vi "Create Arbitrary Waveform.vi"(6 "Arbitrary Numeric Waveform Data":dbl[](array[numeric])=[1000.0, 2000.0, 3000.0, 4000.0, 5000.0, 6000.0, 7000.0, 8000.0], 7 "Waveform Parameters":T1={"Frequency (1000 Hz)"=1000.0, "Amplitude (2.0 Vpp)"=2.0, "DC Offset (0.00 V)"=0.0, "Phase (0.0 degrees)"=0.002} {"Phase (0.0 degrees)" min=-360.0 max=360.0 format="%#.1g"; "DC Offset (0.00 V)" min=-10.0 max=10.0; "Amplitude (2.0 Vpp)" min=0.001 max=20.0 step=1.0 format="%#.3f"; "Frequency (1000 Hz)" min=1e-06 max=160000000.0 step=1.0 format="%#.6g"}, 8 "error in (no error)":errorcluster, 9 "Select Channel (1:Channel 1)":i32(ring)=1 items=["Channel 1"=1, "Channel 2"=2], 10 "Waveform Name (\"wave1\")":string="wave1", 11 "VISA resource name":refnum<visa-resource-name>) -> (0 "error out":errorcluster, 3 "VISA resource name out":refnum<visa-resource-name>)   [LabVIEW 2023, in "Siglent SDG X Series.lvlib"]
doc: "Creates and saves an arbitrary (user-defined) waveform in non-volatile memory, then selects it for output."
uses:
  Siglent SDG X Series.lvlib
  <vilib>/Utility/error.llb/Trim Whitespace One-Sided.vi
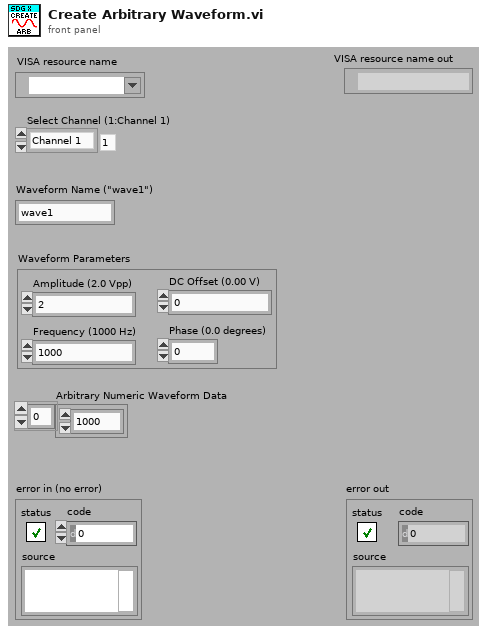
[diagram p1: front panel]
types:
  T1 = cluster{"Frequency (1000 Hz)":dbl, "Amplitude (2.0 Vpp)":dbl, "DC Offset (0.00 V)":dbl, "Phase (0.0 degrees)":dbl}
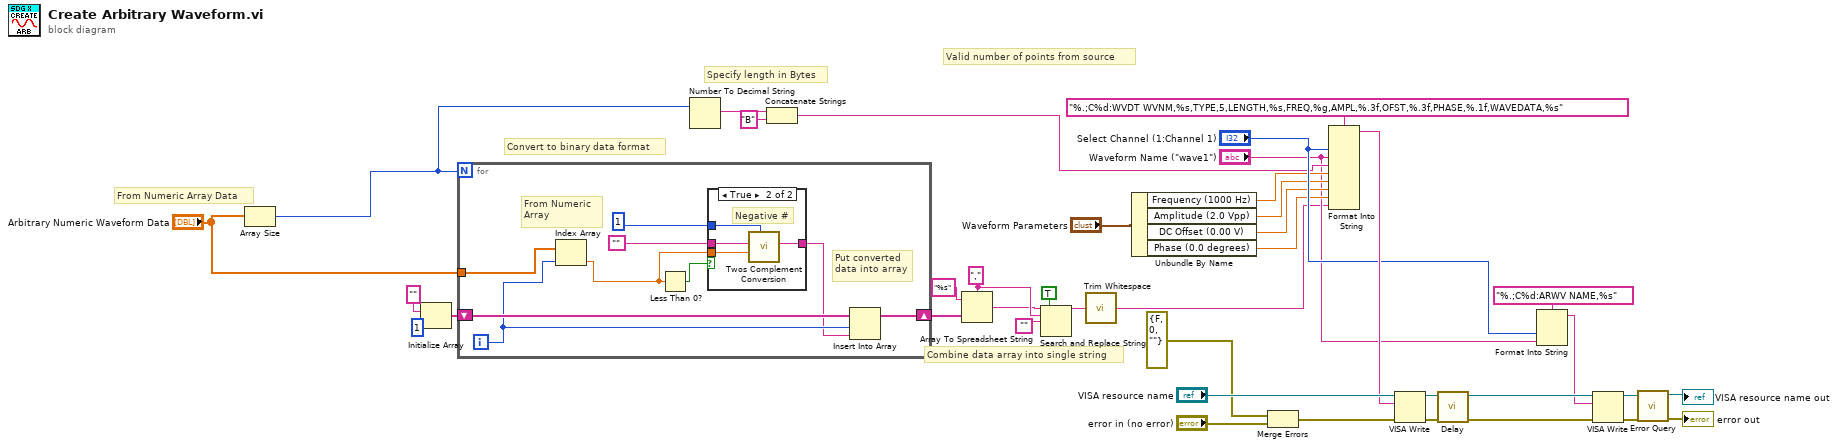
[diagram p0: block diagram]
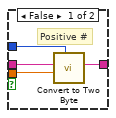
[diagram p2: hidden frame]
diagram:
  w20 = ","
  # "From Numeric Array Data"
  # "Specify length in Bytes"
  # "Combine data array into single string"
  # "Valid number of points from source"
  # "Convert to binary data format"
  n1 = Array Size(array="Arbitrary Numeric Waveform Data") -> (size(s)=w28:i32)
  n2 = Initialize Array("", 1) -> (w24:string[])
  n3 = for {
    N: w28 -> [_]
    tunnel: "Arbitrary Numeric Waveform Data" -> [w44]
    shift-right: [w40] -> w1
    shift-left: w24 -> [w43]
    i -> [w42]
    # "From Numeric\nArray"
    # "Put converted\ndata into array"
    n4 = Index Array(array=w44, index=w42) -> (element=w47:dbl)
    n5 = Less Than 0?(x=w47) -> (x < 0?=w48:bool)
    n6 = case shown="True" w48 {
      tunnel: w47 -> [w49 w54]
      tunnel: [w51 w55] -> w41
      tunnel: "" -> [w52 w56]
      tunnel: u16 1 -> [w50 w53]
      frame False {
        # "Positive #"
        n7 = call "Convert to Two Byte.vi"("Input Method (0:String)"=w50, "Input Number"=w49, "Numeric String"=w52) -> ("Output String"=w51:string)  [unwired: 8 in]
      }
      frame True {
        # "Negative #"
        n8 = call "Twos Complement Conversion.vi"("Input Method (0:String)"=w53, "Input Number"=w54, "Input String"=w56) -> ("Output String"=w55:string)  [unwired: 8 in]
      }
    }
    n9 = Insert Into Array(array=w43, index=w42, new element=w41) -> (w40:string[])
  }
  n10 = Number To Decimal String(number=w28) -> (decimal integer string=w14:string)  [unwired: 1 in]
  n11 = Concatenate Strings(w14, "B" ("string")) -> (w12:string)
  n12 = Array To Spreadsheet String(delimiter (Tab)=w20, array=w1, 3:"%s") -> (spreadsheet string=w17:string)
  n13 = Search and Replace String(replace all?=TRUE, input string=w17, search string=w20, replace string="") -> (result string=w18:string)  [unwired: 4 in, 3 out]
  n14 = call <vilib>:"Trim Whitespace.vi"("string"=w18) -> ("trimmed string"=w2:string)  [unwired: 1 in]
  n15 = Unbundle By Name("Waveform Parameters") -> ("Frequency (1000 Hz)"=w11:dbl, "Amplitude (2.0 Vpp)"=w10:dbl, "DC Offset (0.00 V)"=w9:dbl, "Phase (0.0 degrees)"=w8:dbl)
  n16 = Merge Errors(errorcluster {"status"=FALSE, "code"=0, "source"=""} ("error constant"), "error in (no error)") -> (w30:errorcluster)
  n17 = Format Into String(format string="%.;C%d:WVDT WVNM,%s,TYPE,5,LENGTH,%s,FREQ,%g,AMPL,%.3f,OFST,%.3f,PHASE,%.1f,WAVEDATA,%s", "Select Channel (1:Channel 1)", "Waveform Name (\"wave1\")", w12, w11, w10, w9, w8, w2) -> (resulting string=w33:string)  [unwired: 2 in, 1 out]
  n18 = VISA Write(VISA resource name="VISA resource name", write buffer=w33, error in (no error)=w30) -> (VISA resource name out=w38:refnum<visa-resource-name>, error out=w37:errorcluster)  [unwired: 1 out]
  n19 = call "Delay.vi"("error in (no error)"=w37, "VISA resource name"=w38) -> ("error out"=w35:errorcluster, "VISA resource name out"=w36:refnum<visa-resource-name>)  [unwired: 8 in]
  n20 = Format Into String(format string="%.;C%d:ARWV NAME,%s", "Select Channel (1:Channel 1)", "Waveform Name (\"wave1\")") -> (resulting string=w29:string)  [unwired: 2 in, 1 out]
  n21 = VISA Write(VISA resource name=w36, write buffer=w29, error in (no error)=w35) -> (VISA resource name out=w5:refnum<visa-resource-name>, error out=w6:errorcluster)  [unwired: 1 out]
  n22 = call "Error Query.vi"("error in (no error)"=w6, "VISA resource name"=w5) -> ("error out"=→"error out":errorcluster, "VISA resource name out"=→"VISA resource name out":refnum<visa-resource-name>)  [unwired: 6 in, 2 out]
